vi "Insert VI into SubPanel.vi"(9 "error in":errorcluster, 10 "SubPnl Ref":refnum<vi>, 11 "VI in":refnum<vi>) -> (1 "error out":errorcluster)   [LabVIEW 2023]
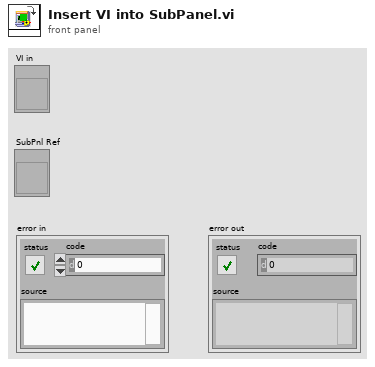
[diagram p1: front panel]
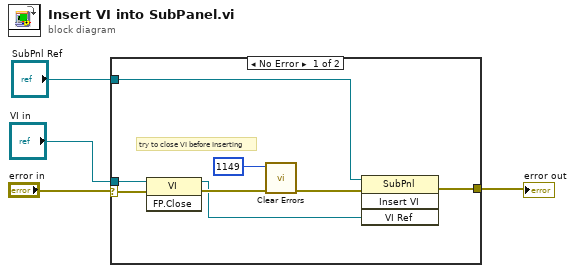
[diagram p0: block diagram]
diagram:
  n1 = case shown="No Error" "error in" {
    selector: "error in" -> [w5 w13]
    tunnel: "VI in" -> [w10 _]
    tunnel: [w8 w13] -> w3
    tunnel: "SubPnl Ref" -> [w6 _]
    frame No Error {
      # "try to close VI before Inserting"
      n2 = invoke class="VI" method="FP.Close"(reference=w10, error in=w5) -> (reference out=w7:refnum<vi>, error out=w11:errorcluster)  [unwired: 1 in, 1 out]
      n3 = call <vilib>:"Clear Errors.vi"("error in (no error)"=w11, "specific error code to clear (0: all)"=1149) -> ("error out"=w9:errorcluster)  [unwired: 4 in, 1 out]
      n4 = invoke on="Invoke Node" class="SubPnl" method="Insert VI"(reference=w6, error in=w9, "VI Ref"=w7) -> (error out=w8:errorcluster)  [unwired: 1 in, 3 out]
    }
    frame Error {
    }
  }
  "error out" <- w3
